vi "CreateNewWizard_Invoke Core.vi"(10 "Wizard":T2, 11 "Cluster":T1) -> (3 "Canceled":bool)   [LabVIEW 2023, in "Add Async Methods Actor.lvlib"]
uses:
  Add Async Methods Actor.lvlib
  <resource>/Framework/Providers/API/ItemRef.ctl
  <resource>/Framework/Providers/API/mxLvNIIM.ctl
  Localized Strings.vi
  AFPP Shared/AFPP Shared.lvlib
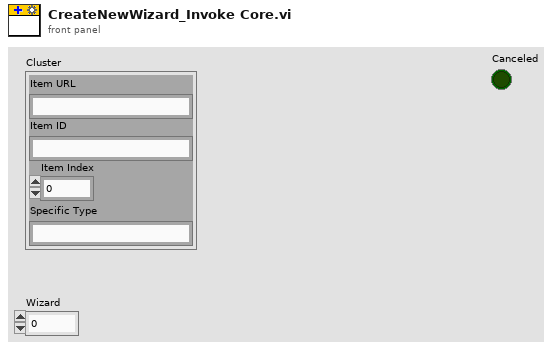
[diagram p1: front panel]
types:
  T1 = typedef "mxLvNIIM.ctl" = cluster{"Item URL":string, "Item ID":string, "Item Index":i32, "Specific Type":string}
  T2 = typedef "ItemRef.ctl" = u64
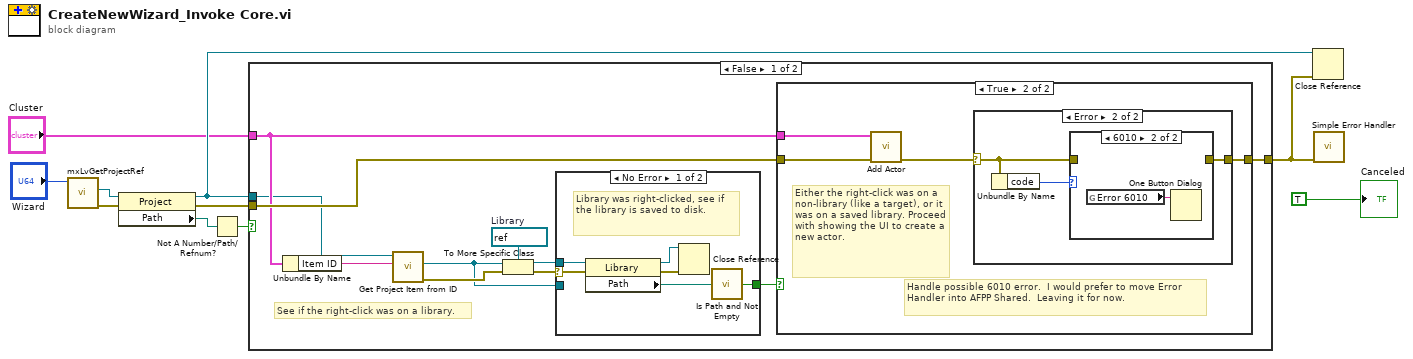
[diagram p0: block diagram]
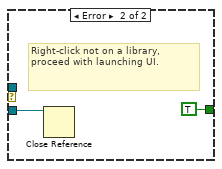
[diagram p2: hidden frame]
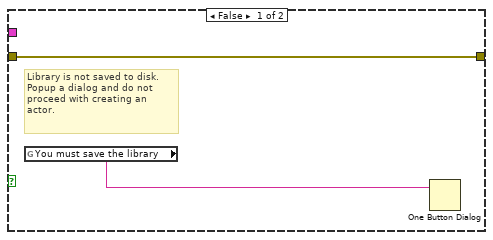
[diagram p3: hidden frame]
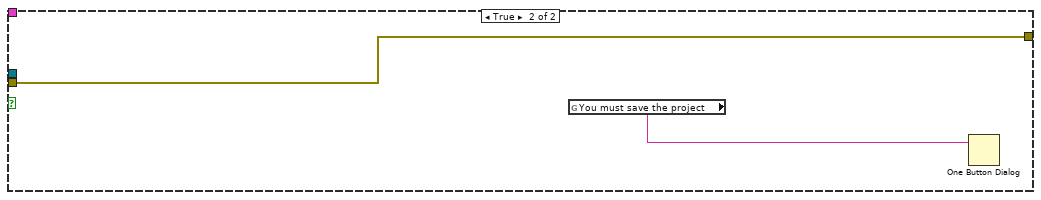
[diagram p6: hidden frame]
diagram:
  n1 = call <resource>:"mxLvGetProjectRef.vi"("Item"="Wizard") -> ("error out"=w4:errorcluster, "Project Refnum"=w3:refnum<vi>)  [unwired: 8 in, 1 out]
  n2 = property class="Project"(reference=w3, error in=w4) -> (reference out=w10:refnum<vi>, error out=w7:errorcluster, "Path"=w5:path)
  n3 = Not A Number/Path/Refnum?(number/path/refnum=w5) -> (NaN/Path/Refnum?=w6:bool)
  n4 = case shown="False" w6 {
    tunnel: [w21 w43] -> w9
    tunnel: "Cluster" -> [w15 _]
    tunnel: w7 -> [w20 w43]
    tunnel: w10 -> [w14 _]
    frame False {
      w19 = refnum<vi> refnum  # Library
      # "See if the right-click was on a library."
      n5 = Unbundle By Name(w15) -> ("Item ID"=w13:string)
      n6 = call "Get Project Item from ID.vi"("Item ID"=w13, "Project in"=w14) -> ("error out"=w12:errorcluster, "Project Item"=w11:refnum<vi>)  [unwired: 7 in, 1 out]
      n7 = To More Specific Class(target class=w19, reference=w11, error in=w12) -> (specific class reference=w18:refnum<vi>, error out=w17:errorcluster)
      n8 = case shown="No Error" w17 {
        selector: w17 -> [w26 _]
        tunnel: w18 -> [w27 _]
        tunnel: [w22 TRUE ("Is Path and Not Empty?")] -> w16
        tunnel: w11 -> [_ w28]
        frame No Error {
          # "Library was right-clicked, see if the library is saved to disk."
          n9 = property class="Library"(reference=w27, error in=w26) -> (reference out=w24:refnum<vi>, error out=w25:errorcluster, "Path"=w23:path)
          n10 = Close Reference(reference=w24, error in (no error)=w25) -> ()  [unwired: 1 out]
          n11 = call <vilib>:"Is Path and Not Empty.vi"("path"=w23) -> ("Is Path and Not Empty?"=w22:bool)  [unwired: 4 in]
        }
        frame Error {
          # "Right-click not on a library, proceed with launching UI."
          n12 = Close Reference(reference=w28) -> ()  [unwired: 1 in, 1 out]
        }
      }
      n13 = case shown="True" w16 {
        tunnel: [w31 w32] -> w21
        tunnel: w15 -> [_ w35]
        tunnel: w20 -> [w31 w34]
        frame False {
          # "Library is not saved to disk. Popup a dialog and do not proceed with creating an actor."
          n14 = global read "Localized Strings.vi" "You must save the library"() -> (w30:string)
          n15 = One Button Dialog(message=w30) -> ()  [unwired: 1 in, 1 out]
        }
        frame True {
          # "Handle possible 6010 error.  I would prefer to move Error Handler into AFPP Shared.  Leaving it for now."
          # "Either the right-click was on a non-library (like a target), or it was on a saved library. Proceed with showing the UI to create a new actor."
          n16 = call "Add Actor.vi"("error in"=w34, "Target Item"=w35) -> ("error out"=w33:errorcluster)  [unwired: 9 in]
          n17 = case shown="Error" w33 {
            selector: w33 -> [w36 w37]
            tunnel: [w36 w39] -> w32
            frame No Error {
            }
            frame Error {
              n18 = Unbundle By Name(w37) -> ("code"=w38:i32)
              n19 = case shown="6010" w38 {
                tunnel: [w40 _] -> w39
                tunnel: w37 -> [w40 _]
                frame Default {
                }
                frame 6010 {
                  n20 = global read "Localized Strings.vi" "Error 6010"() -> (w41:string)
                  n21 = One Button Dialog(message=w41) -> ()  [unwired: 1 in, 1 out]
                }
              }
            }
          }
        }
      }
    }
    frame True {
      n22 = global read "Localized Strings.vi" "You must save the project"() -> (w42:string)
      n23 = One Button Dialog(message=w42) -> ()  [unwired: 1 in, 1 out]
    }
  }
  n24 = Close Reference(reference=w10, error in (no error)=w9) -> ()  [unwired: 1 out]
  n25 = call <vilib>:"Simple Error Handler.vi"("error in (no error)"=w9) -> ()  [unwired: 4 in, 5 out]
  "Canceled" <- TRUE ("Canceled")
